vi "FlipGreyscale.vi"(7 "Flip Mode (Default: X-Axis)":T1, 8 "error in (no error)":errorcluster, 10 "Greyscale Destination Image":refnum<data-value>, 11 "Greyscale Source Image":refnum<data-value>) -> (0 "error out":errorcluster, 3 "Greyscale Destination Image (duplicate)":refnum<data-value>)   [LabVIEW 2020, in "g_ar_toolkit.image.lvlib"]
uses:
  g_ar_toolkit.image.lvlib
  348de330-10c9-445f-8d54-7780e9118077.vi
  Flip Mode.ctl
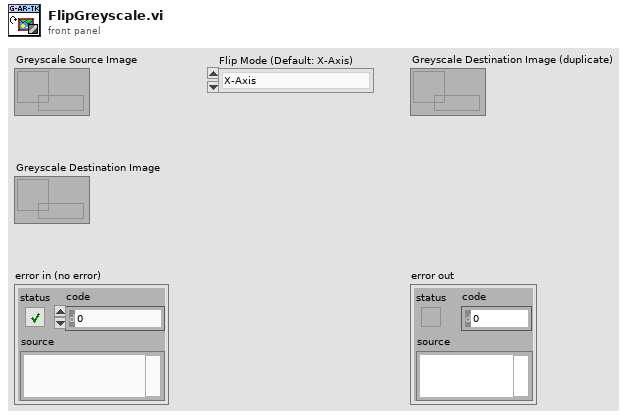
[diagram p1: front panel]
types:
  T1 = typedef "g_ar_toolkit.image.lvlib/Flip Mode.ctl" = enum16{"X-Axis", "Y-Axis", "X and Y Axes"}
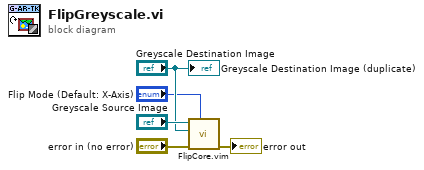
[diagram p0: block diagram]
diagram:
  n1 = call "FlipCore.vim"("Flip Mode"="Flip Mode (Default: X-Axis)", "error in (no error)"="error in (no error)", "Destination Image"="Greyscale Destination Image", "Source Image"="Greyscale Source Image") -> ("error out"=→"error out":errorcluster)  [unwired: 7 in]
  "Greyscale Destination Image (duplicate)" <- "Greyscale Destination Image"
